vi "Edit Sensor Calibration Table.vi.vi"(7 "Table Name (0)":string="0", 8 "error in (no error)":errorcluster, 9 "Calibration Data (0)":string="0", 10 "Frequency Data (0)":string="0", 11 "VISA resource name":refnum<visa-resource-name>) -> (0 "error out":errorcluster, 3 "VISA resource name out":refnum<visa-resource-name>)   [LabVIEW 2011, in "Agilent N432A.lvlib"]
doc: "Edits a specific sensor calibration table."
uses:
  <instrlib>/Agilent N432A/Agilent N432A.lvlib
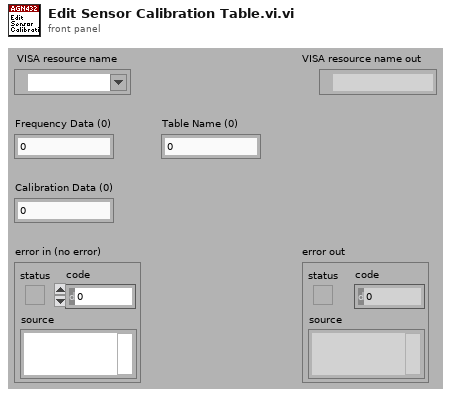
[diagram p1: front panel]
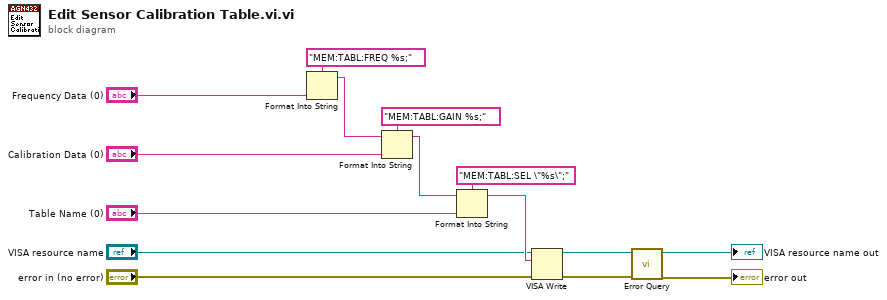
[diagram p0: block diagram]
diagram:
  n1 = Format Into String(format string="MEM:TABL:FREQ %s;", "Frequency Data (0)") -> (resulting string=w13:string)  [unwired: 2 in, 1 out]
  n2 = Format Into String(format string="MEM:TABL:GAIN %s;", initial string=w13, "Calibration Data (0)") -> (resulting string=w10:string)  [unwired: 1 in, 1 out]
  n3 = Format Into String(format string="MEM:TABL:SEL \"%s\";", initial string=w10, "Table Name (0)") -> (resulting string=w7:string)  [unwired: 1 in, 1 out]
  n4 = VISA Write(VISA resource name="VISA resource name", write buffer=w7, error in (no error)="error in (no error)") -> (VISA resource name out=w4:refnum<visa-resource-name>, error out=w3:errorcluster)  [unwired: 1 out]
  n5 = call <instrlib>:"Error Query.vi"("error in (no error)"=w3, "VISA resource name"=w4) -> ("error out"=→"error out":errorcluster, "VISA resource name out"=→"VISA resource name out":refnum<visa-resource-name>)  [unwired: 6 in, 2 out]
